vi "Configure Dialog.vi"(7 "Data in":path, 11 "Persistent Path Selector in":refnum<class "MGI Persistent Path Selector.lvclass">) -> (2 "Changed?":bool, 3 "Persistent Path Selector out":refnum<class "MGI Persistent Path Selector.lvclass">, 5 "Data out":path)   [LabVIEW 2016, in "MGI Persistent Path Selector.lvclass"]
uses:
  <userlib>/_MGI/User Interface/Path Selector XControl/Class Hierarchy/Persistent Path Selector/MGI Persistent Path Selector.lvclass
  <userlib>/_MGI/User Interface/Path Selector XControl/Control Style Enum.ctl
  <userlib>/_MGI/User Interface/Path Selector XControl/MGI Path Selector.xctl
panel:
  in  "Section":string
  in  "INI File":path caption="Config File is a MGI RWA file used to store the last path"
  in  "Control Style":T1 caption="Control Style of File Selector"
  in  "Filter":string(combo) caption="Filter: Type in desired filter or select existing option below:"
  in  "Browse Option":bool
  in  "Explore Option":bool
  in  "Allow New":bool
  in  "Recursive List":bool
  in  "Path":path caption="Initial Path"
  in  "Done":bool
  # "This dialog allows configuration of the File Selector.\nThe file selector is a combo box that shows files from a directory and allows the user to select a file.    The directory containing the files (file directory) is typically the folder containing the file last selected by the user.  The File Selector remembers which file is selected by the user by saving this information to a file."
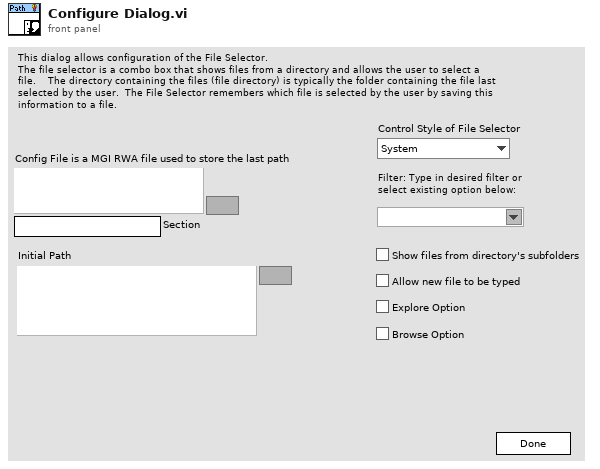
[diagram p1: front panel]
types:
  T1 = typedef "MGI Path Selector.xctl/Control Style Enum.ctl" = enum16{"System", "Modern", "Classic", "Silver"}
  T2 = enum16{"Left Button", "Center Button", "Right Button", "Window Close"}
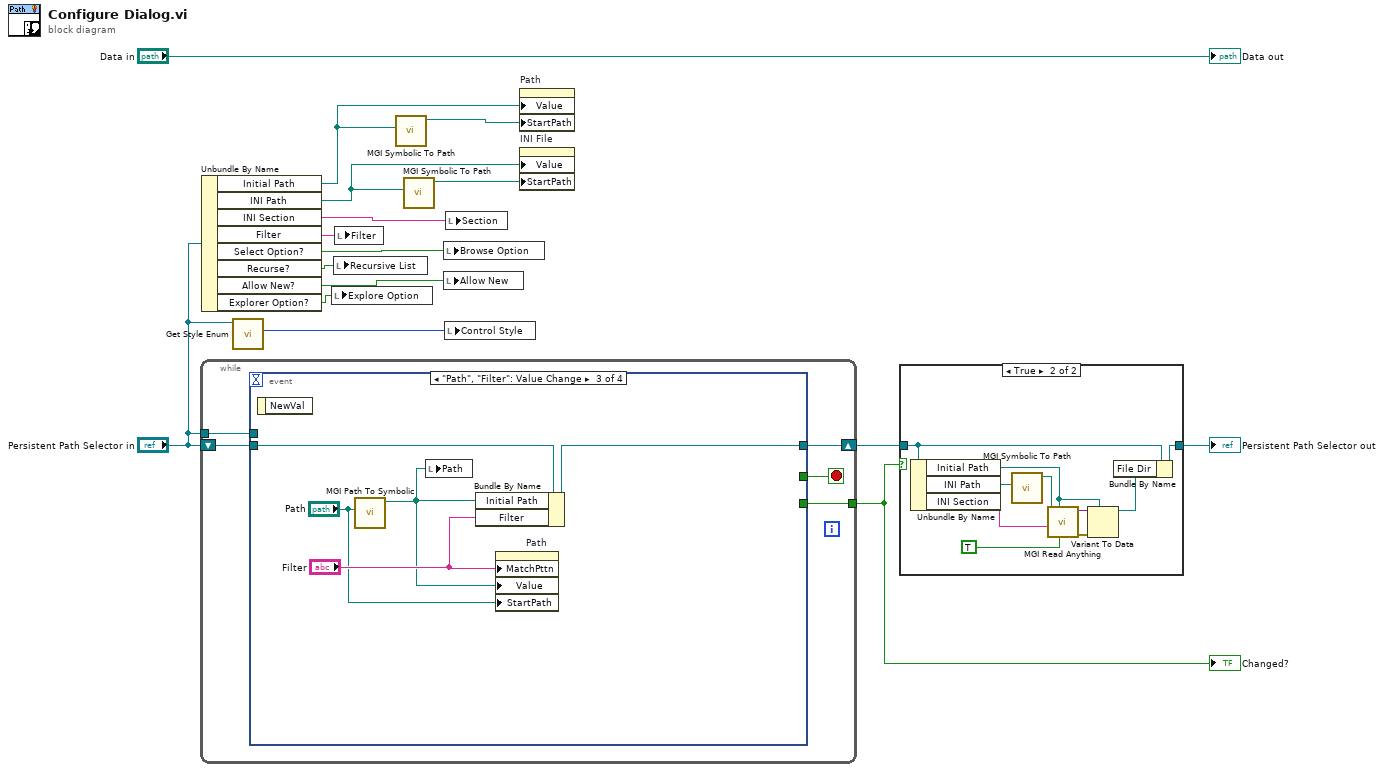
[diagram p0: block diagram]
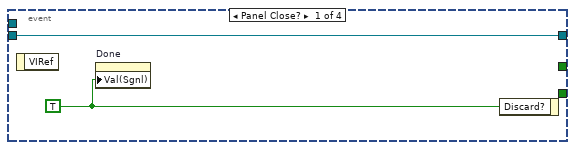
[diagram p3: hidden frame]
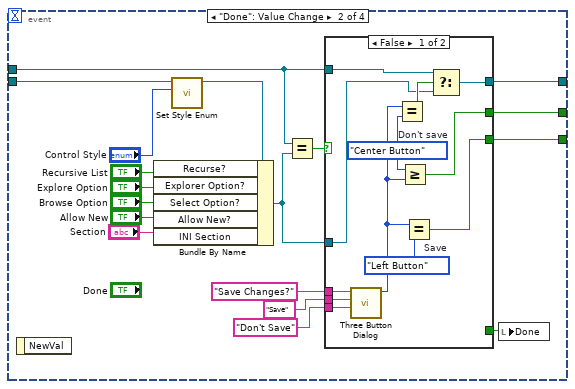
[diagram p4: hidden frame]
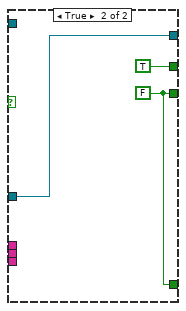
[diagram p5: hidden frame]
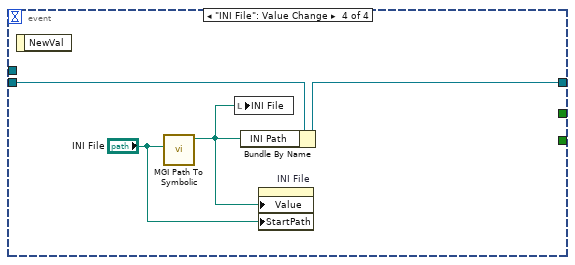
[diagram p6: hidden frame]
diagram:
  n1 = while {
    shift-right: [w17] -> w6
    shift-left: "Persistent Path Selector in" -> [w21]
    tunnel: "Persistent Path Selector in" -> [w20]
    tunnel: [w18] -> w7
    stop <- w19 stop-if-true
    n2 = event shown="[2] \"Path\", \"Filter\": Value Change" {
      selector: _ -> [_ _ _ _]
      dyn-events: _ -> [_ _ _ _]
      timeout: _ -> [_ _ _ _]
      tunnel: w21 -> [w23 w27 w61 w65]
      tunnel: w20 -> [_ w36 _ _]
      tunnel: [_ w31 _ _] -> w19
      tunnel: [_ w30 _ _] -> w18
      tunnel: [w23 w32 w60 w64] -> w17
      event Panel Close? {
        w22 = TRUE ("Discard?")
        n3 = event-data() -> ()  [unwired: 1 in, 1 out]
        n4 = property on="Done" class="Bool (strict)"("Val(Sgnl)"=w22) -> ()  [unwired: 2 in, 2 out]
        n5 = event-data("Discard?"=w22) -> ()  [unwired: 1 in, 1 out]
      }
      event "Done": Value Change {
        n6 = event-data() -> ()  [unwired: 1 in, 1 out]
        n7 = call-dynamic "Set Style Enum.vi"("Control Style"="Control Style", "Path Selector in"=w27) -> ("Path Selector out"=w26:refnum<class "MGI Persistent Path Selector.lvclass">)  [unwired: 9 in]
        n8 = Bundle By Name(cluster=w26, "Recurse?"="Recursive List", "Explorer Option?"="Explore Option", "Select Option?"="Browse Option", "Allow New?"="Allow New", "INI Section"="Section") -> (w28:refnum<class "MGI Persistent Path Selector.lvclass">)
        n9 = Equal?(x=w36, y=w28) -> (x = y?=w37:bool)
        n10 = case shown="False" w37 {
          tunnel: w36 -> [w47 _]
          tunnel: "Save Changes?" ("message") -> [w53 _]
          tunnel: "Save" ("Left Button Text (\"Yes\")") -> [w52 _]
          tunnel: "Don't Save" ("Center Button Text (\"No\")") -> [w51 _]
          tunnel: [w46 w54] -> w32
          tunnel: [w50 TRUE] -> w31
          tunnel: [w43 w55] -> w30
          tunnel: [_ w55] -> w29
          tunnel: w28 -> [w42 w54]
          frame False {
            w44 = T2."Left Button"  # Save
            w49 = T2."Center Button"  # Don't save
            n11 = call <vilib>:"Three Button Dialog.vi"("Center Button Text (\"No\")"=w51, "Left Button Text (\"Yes\")"=w52, "message"=w53) -> ("Which Button?"=w45:T2)  [unwired: 8 in]
            n12 = Equal?(x=w45, y=w49) -> (x = y?=w48:bool)
            n13 = Greater Or Equal?(x=w49, y=w45) -> (x >= y?=w50:bool)
            n14 = Equal?(x=w45, y=w44) -> (x = y?=w43:bool)
            n15 = Select(t=w47, s=w48, f=w42) -> (s? t:f=w46:refnum<class "MGI Persistent Path Selector.lvclass">)
          }
          frame True {
            w55 = FALSE
          }
        }
        n16 = local write "Done"(w29) -> ()
      }
      event "Path", "Filter": Value Change {
        n17 = event-data() -> ()  [unwired: 1 in, 1 out]
        n18 = call <userlib>:"MGI Path To Symbolic.vi"("Path"="Path") -> ("Symbolic Path"=w57:path)  [unwired: 8 in, 2 out]
        n19 = local write "Path"(w57) -> ()
        n20 = Bundle By Name(cluster=w61, "Initial Path"=w57, "Filter"="Filter") -> (w60:refnum<class "MGI Persistent Path Selector.lvclass">)
        n21 = property on="Path" class="Path"("MatchPttn"="Filter", "Value"=w57, "StartPath"="Path") -> ()  [unwired: 2 in, 2 out]
      }
      event "INI File": Value Change {
        n22 = event-data() -> ()  [unwired: 1 in, 1 out]
        n23 = call <userlib>:"MGI Path To Symbolic.vi"("Path"="INI File") -> ("Symbolic Path"=w62:path)  [unwired: 8 in, 2 out]
        n24 = local write "INI File"(w62) -> ()
        n25 = Bundle By Name(cluster=w65, "INI Path"=w62) -> (w64:refnum<class "MGI Persistent Path Selector.lvclass">)
        n26 = property on="INI File" class="Path"("Value"=w62, "StartPath"="INI File") -> ()  [unwired: 2 in, 2 out]
      }
    }
  }
  "Changed?" <- w7
  n27 = Unbundle By Name("Persistent Path Selector in") -> ("Initial Path"=w4:path, "INI Path"=w2:path, "INI Section"=w13:string, "Filter"=w14:string, "Select Option?"=w12:bool, "Recurse?"=w11:bool, "Allow New?"=w10:bool, "Explorer Option?"=w15:bool)
  n28 = call-dynamic "Get Style Enum.vi"("Path Selector in"="Persistent Path Selector in") -> ("Control Style"=w8:T1)  [unwired: 10 in]
  n29 = local write "Explore Option"(w15) -> ()
  n30 = local write "Recursive List"(w11) -> ()
  n31 = local write "Filter"(w14) -> ()
  n32 = call <userlib>:"MGI Symbolic To Path.vi"("Symbolic Path"=w4) -> ("Path"=w3:path)  [unwired: 8 in, 2 out]
  n33 = call <userlib>:"MGI Symbolic To Path.vi"("Symbolic Path"=w2) -> ("Path"=w1:path)  [unwired: 8 in, 2 out]
  n34 = local write "Browse Option"(w12) -> ()
  n35 = local write "Allow New"(w10) -> ()
  n36 = local write "Control Style"(w8) -> ()
  n37 = local write "Section"(w13) -> ()
  n38 = property on="Path" class="Path"("Value"=w4, "StartPath"=w3) -> ()  [unwired: 2 in, 2 out]
  n39 = property on="INI File" class="Path"("Value"=w2, "StartPath"=w1) -> ()  [unwired: 2 in, 2 out]
  n40 = case shown="True" w7 {
    tunnel: w6 -> [w66 w71]
    tunnel: [w66 w70] -> w5
    frame False {
    }
    frame True {
      n41 = Unbundle By Name(w71) -> ("Initial Path"=w74:path, "INI Path"=w68:path, "INI Section"=w73:string)
      n42 = call <userlib>:"MGI Symbolic To Path.vi"("Symbolic Path"=w68) -> ("Path"=w67:path)  [unwired: 8 in, 2 out]
      n43 = call <userlib>:"MGI Read Anything.vi"("Use Supplied (F: Use Default)"=TRUE, "Type of Anything"=w74, "Section Name (Name of \"Type of Anything\")"=w73, "Path (dialog)"=w67) -> ("Error Out"=w76:errorcluster, "Anything"=w75:variant)  [unwired: 4 in, 2 out]
      n44 = Variant To Data(error in=w76, type=w74, Variant=w75) -> (data=w69:path)  [unwired: 1 out]
      n45 = Bundle By Name(cluster=w71, "File Dir"=w69) -> (w70:refnum<class "MGI Persistent Path Selector.lvclass">)
    }
  }
  "Persistent Path Selector out" <- w5
  "Data out" <- "Data in"
